vi "Logic.vi"(8 "Switch 4":bool, 9 "Switch 3":bool, 10 "Switch 2":bool, 11 "Switch 1":bool) -> (2 "x != 0?":bool, 3 "String":string)   [LabVIEW 2012]
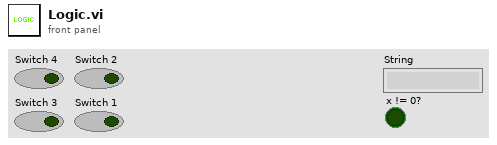
[diagram p1: front panel]
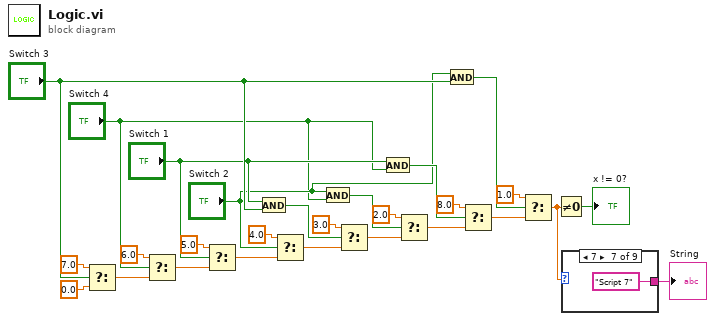
[diagram p0: block diagram]
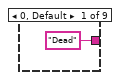
[diagram p2: hidden frame]
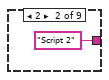
[diagram p3: hidden frame]
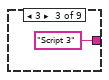
[diagram p4: hidden frame]
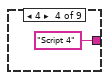
[diagram p5: hidden frame]
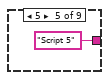
[diagram p6: hidden frame]
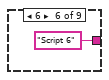
[diagram p7: hidden frame]
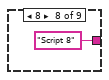
[diagram p8: hidden frame]
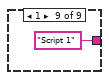
[diagram p9: hidden frame]
diagram:
  n1 = Select(t=7.0, s="Switch 3", f=0.0) -> (s? t:f=w6:dbl)
  n2 = Select(t=6.0, s="Switch 4", f=w6) -> (s? t:f=w26:dbl)
  n3 = Select(t=5.0, s="Switch 1", f=w26) -> (s? t:f=w24:dbl)
  n4 = And(x="Switch 1", y="Switch 3") -> (x .and. y?=w17:bool)
  n5 = Select(t=4.0, s="Switch 2", f=w24) -> (s? t:f=w22:dbl)
  n6 = And(x="Switch 2", y="Switch 4") -> (x .and. y?=w12:bool)
  n7 = Select(t=3.0, s=w17, f=w22) -> (s? t:f=w18:dbl)
  n8 = And(x="Switch 1", y="Switch 4") -> (x .and. y?=w15:bool)
  n9 = Select(t=2.0, s=w12, f=w18) -> (s? t:f=w20:dbl)
  n10 = And(x="Switch 2", y="Switch 3") -> (x .and. y?=w14:bool)
  n11 = Select(t=8.0, s=w15, f=w20) -> (s? t:f=w9:dbl)
  n12 = Select(t=1.0, s=w14, f=w9) -> (s? t:f=w5:dbl)
  n13 = Not Equal To 0?(x=w5) -> (x != 0?=→"x != 0?":bool)
  n14 = case shown="7" w5 {
    tunnel: ["Dead" "Script 2" "Script 3" "Script 4" "Script 5" "Script 6" "Script 7" "Script 8" "Script 1"] -> w10
    frame 0, Default {
    }
    frame 2 {
    }
    frame 3 {
    }
    frame 4 {
    }
    frame 5 {
    }
    frame 6 {
    }
    frame 7 {
    }
    frame 8 {
    }
    frame 1 {
    }
  }
  "String" <- w10
